vi "状态告警区_选择.vi"(11 "data":u16[](array[numeric]) format="%04xH") -> (2 "状态告警区 2":T1, 3 "状态告警区":T2)   [LabVIEW 2016, in "斯坦道氨氮.lvlib"]
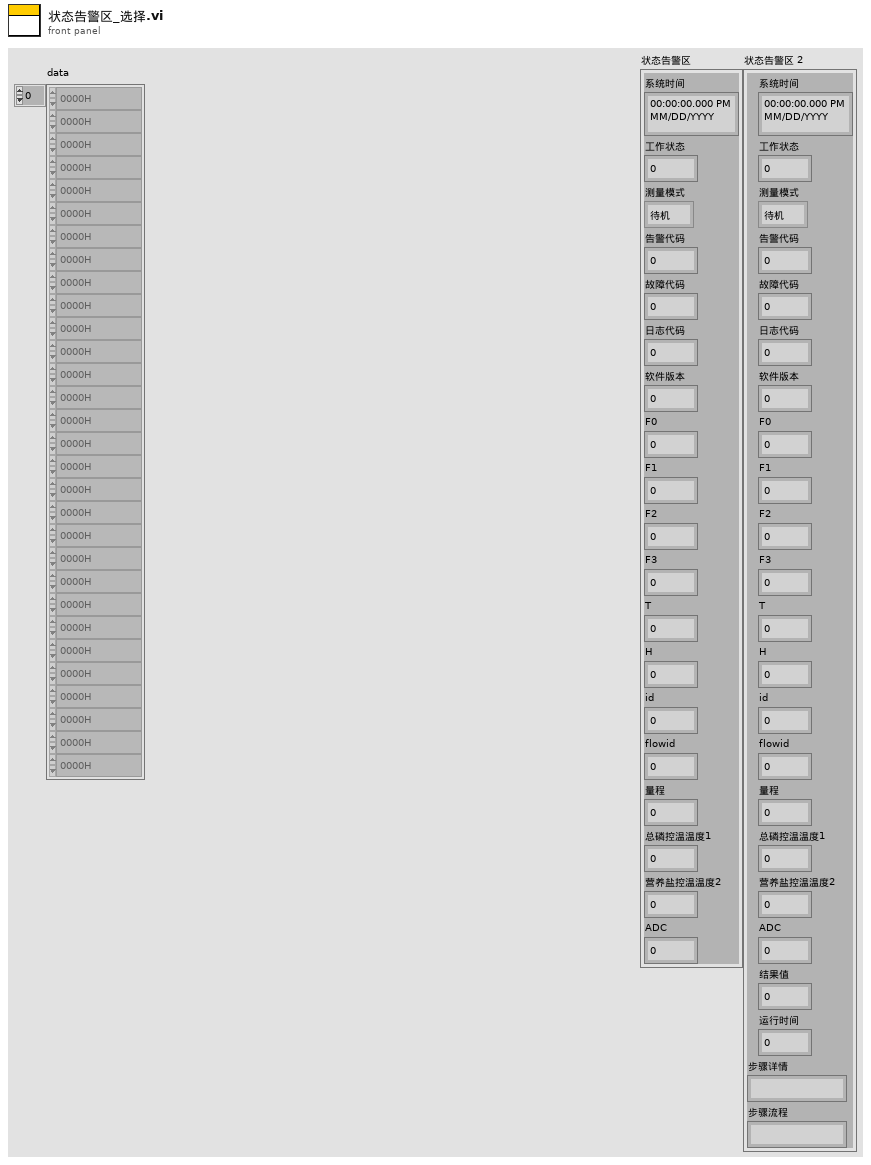
[diagram p1: front panel]
types:
  T1 = cluster{"系统时间":timestamp, "工作状态":u16, "测量模式":enum16{"待机", "连续模式", "周期模式", "定点模式", "受控模式", "手动模式"}, "告警代码":u16, "故障代码":u16, "日志代码":u16, "软件版本":u16, "F0":sgl, "F1":sgl, "F2":sgl, "F3":sgl, "T":sgl, "H":sgl, "id":u16, "flowid":u16, "量程":u16, "总磷控温温度1":sgl, "营养盐控温温度2":sgl, "ADC":sgl, "结果值":sgl, "运行时间":u16, "步骤详情":string, "步骤流程":string}
  T2 = cluster{"系统时间":timestamp, "工作状态":u16, "测量模式":enum16{"待机", "连续模式", "周期模式", "定点模式", "受控模式", "手动模式"}, "告警代码":u16, "故障代码":u16, "日志代码":u16, "软件版本":u16, "F0":sgl, "F1":sgl, "F2":sgl, "F3":sgl, "T":sgl, "H":sgl, "id":u16, "flowid":u16, "量程":u16, "总磷控温温度1":sgl, "营养盐控温温度2":sgl, "ADC":sgl}
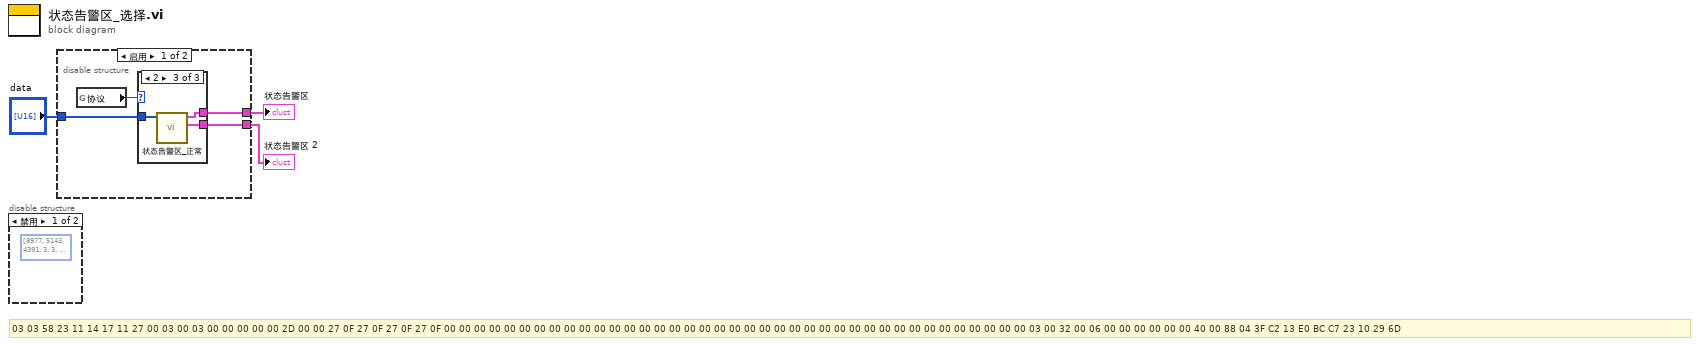
[diagram p0: block diagram]
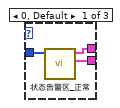
[diagram p2: hidden frame]
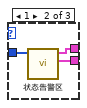
[diagram p3: hidden frame]
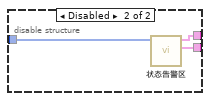
[diagram p4: hidden frame]
diagram:
  # "03 03 58 23 11 14 17 11 27 00 03 00 03 00 00 00 00 00 2D 00 00 27 0F 27 0F 27 0F 27 0F 00 00 00 00 00 00 00 00 00 00 00 00 00 00 00 00 00 00 00 00 00 00 00 00 00 00 00 00 00 00 00 00 00 00 00 00 00 00 00 03 00 32 00 06 00 00 00 00 00 00 40 00 88 04 3F C2 13 E0 BC C7 23 10 29 6D"
  n1 = disable-structure shown="禁用" {
    frame Disabled {
      (unwired) u32[] [8977, 5143, 4391, 3, 3, 0, 0, 45, 0, 9999, 9999, 9999, 9999, 0, 0, 0, 0, 0, 0, 0, 0, 0, 0, 0, 0, 0, 0, 0, 0, 0, 0, 0, 3, 50, 6, 0, 0, 0, 16384, 34820, 16322, 5088, 48327, 8976, 10605] ("数组")
    }
    frame Enabled {
    }
  }
  n2 = disable-structure shown="启用" {
    disable-tunnel: "data" -> [w7 w19]
    disable-tunnel: [w6 w18] -> w2
    disable-tunnel: [w5 w17] -> w1
    frame Enabled {
      n3 = global read "总磷总氮断电保存全局变量.vi" "协议"() -> (w4:u16)
      n4 = case shown="2" w4 {
        tunnel: w7 -> [w10 w13 w16]
        tunnel: [w9 w12 w15] -> w6
        tunnel: [w8 w11 w14] -> w5
        frame 0, Default {
          n5 = call "状态告警区_正常.vi"("数组"=w10) -> ("状态告警区 2"=w8:T1, "状态告警区"=w9:T2)  [unwired: 9 in]
        }
        frame 1 {
          n6 = call "状态告警区.vi"("数组"=w13) -> ("状态告警区 2"=w11:T1, "状态告警区"=w12:T2)  [unwired: 9 in]
        }
        frame 2 {
          n7 = call "状态告警区_正常.vi"("数组"=w16) -> ("状态告警区 2"=w14:T1, "状态告警区"=w15:T2)  [unwired: 9 in]
        }
      }
    }
    frame Disabled {
      n8 = call "状态告警区.vi"("数组"=w19) -> ("状态告警区 2"=w17:T1, "状态告警区"=w18:T2)  [unwired: 9 in]
    }
  }
  "状态告警区" <- w2
  "状态告警区 2" <- w1
